vi "Initial Scan for Period Greater Than 1S.vi"(3 "Period (s)":dbl=600.0 caption="周期 (s)" format="%#_13g") -> (0 "Period (scan)":i64 caption="周期 (scan)", 1 "t0 (scan)":i64 caption="起始时间 (scan)")   [LabVIEW 2015]
uses:
  Globals/Global - Monitoring Variables.vi
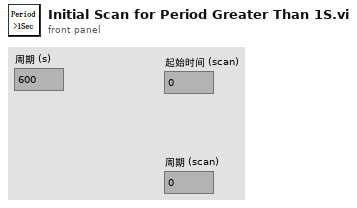
[diagram p1: front panel]
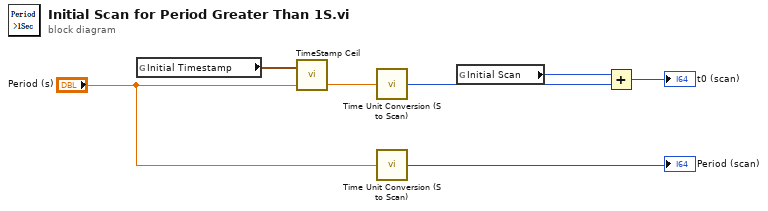
[diagram p0: block diagram]
diagram:
  n1 = global read "Global - Monitoring Variables.vi" "Initial Timestamp"() -> (w7:timestamp)
  n2 = call "TimeStamp Ceil.vi"("base (s)"="Period (s)", "timestamp input"=w7) -> ("time diff (s)"=w4:dbl)  [unwired: 1 out]
  n3 = call "Time Unit Conversion (S to Scan).vi"("time duration (s)"=w4) -> ("time duration (scan)"=w3:i64)
  n4 = call "Time Unit Conversion (S to Scan).vi"("time duration (s)"="Period (s)") -> ("time duration (scan)"=→"Period (scan)":i64)
  n5 = global read "Global - Monitoring Variables.vi" "Initial Scan"() -> (w6:i64)
  n6 = Add(x=w6, y=w3) -> (x+y=→"t0 (scan)":i64)
